vi "ConfigInstr.vi"(6 "InstrumentName":string, 7 "VisaRessIn":refnum<visa-resource-name>, 8 "error in (no error)":errorcluster caption="entrée d'erreur (pas d'erreur)", 9 "FirstClassInst":bool, 10 "Function":string, 11 "GenData In":refnum<class "AppliedMotionDrive.lvclass"> caption="DNL_LabVIEW Object in") -> (0 "error out":errorcluster caption="sortie d'erreur", 3 "GenData Out":refnum<class "AppliedMotionDrive.lvclass"> caption="DNL_LabVIEW Object out")   [LabVIEW 2019, in "AppliedMotionDrive.lvclass"]
uses:
  AppliedMotionDrive.lvclass
  C:/Programmes Labview/LabscanV1A/DevicesClass/BaseDevice/BaseDevice.lvclass
  AppliedMotionDrive_Func.ctl
  AppliedMotionDrive.lvclass/AppliedMotionDrive.ctl
  BaseDevice/BaseDevice.lvclass/BaseDevice.ctl
  BaseDevice/Accessor/SetShowInstrNm.vi
  BaseDevice/Accessor/SetInstrParam.vi
panel:
  in  "DefaultDev_Func":T1
  out "VisaRessOut":refnum<visa-resource-name>
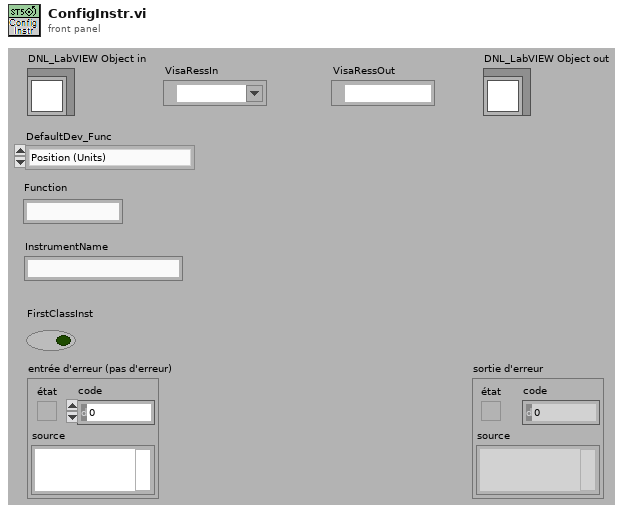
[diagram p1: front panel]
types:
  T1 = typedef "AppliedMotionDrive.lvclass/AppliedMotionDrive_Func.ctl" = enum16{"Position (Units)", "FilterWheel (Id)"}
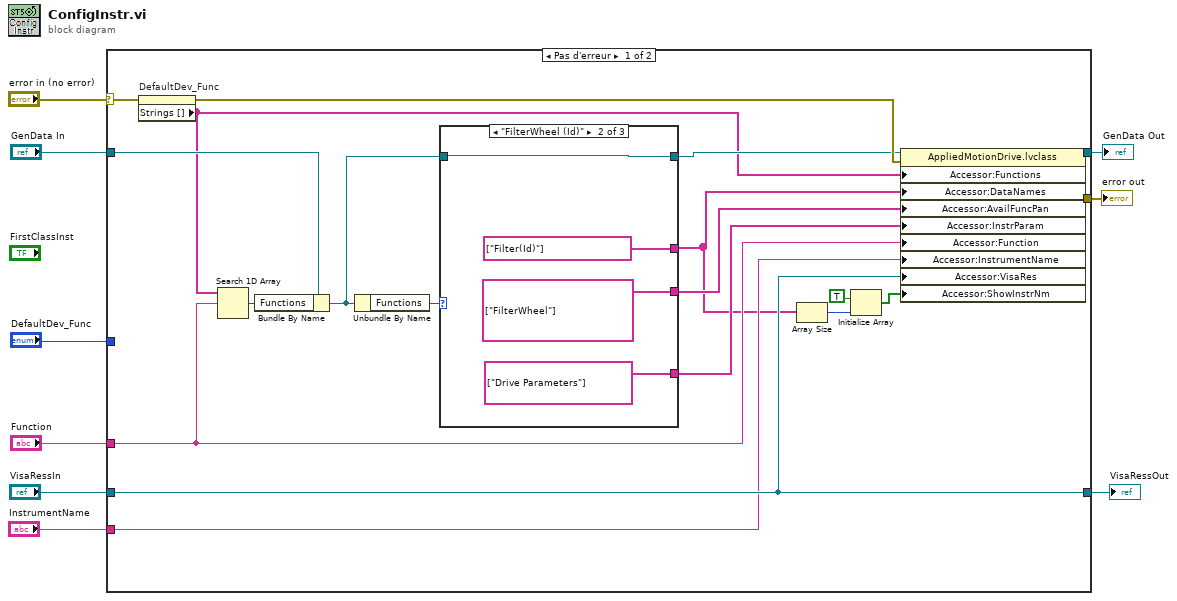
[diagram p0: block diagram]
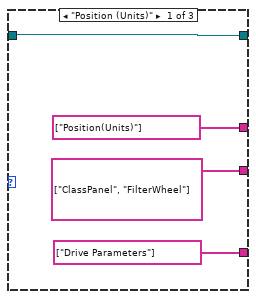
[diagram p2: hidden frame]
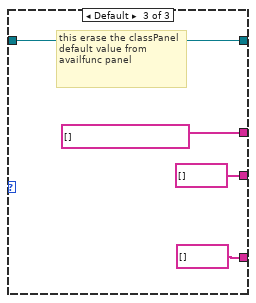
[diagram p3: hidden frame]
diagram:
  n1 = case shown="Pas d'erreur" "error in (no error)" {
    selector: "error in (no error)" -> [w24 w43]
    tunnel: [w28 w43] -> w8
    tunnel: "GenData In" -> [w19 w42]
    tunnel: [w27 w42] -> w6
    tunnel: "DefaultDev_Func" -> [_ _]
    tunnel: "Function" -> [w15 _]
    tunnel: "InstrumentName" -> [w17 _]
    tunnel: "VisaRessIn" -> [w20 w41]
    tunnel: [w20 w41] -> w1
    frame No Error {
      n2 = property on="DefaultDev_Func" class="Énum (strict)"(error in=w24) -> (error out=w23:errorcluster, "Strings []"=w16:string[])  [unwired: 1 in, 1 out]
      n3 = Search 1D Array(1D array=w16, element=w15) -> (index of element=w25:i32)  [unwired: 1 in]
      n4 = Bundle By Name(cluster=w19, "Functions"=w25) -> (w22:refnum<class "AppliedMotionDrive.lvclass">)
      n5 = Unbundle By Name(w22) -> ("Functions"=w26:T1)
      n6 = case shown="\"FilterWheel (Id)\"" w26 {
        tunnel: [string[] ["Position(Units)"] string[] ["Filter(Id)"] string[] []] -> w10
        tunnel: w22 -> [w32 w36 w39]
        tunnel: [w32 w36 w39] -> w21
        tunnel: [string[] ["ClassPanel", "FilterWheel"] string[] ["FilterWheel"] string[] []] -> w18
        tunnel: [string[] ["Drive Parameters"] ("InstrParam") string[] ["Drive Parameters"] ("InstrParam") string[] []] -> w14
        frame "Position (Units)" {
        }
        frame "FilterWheel (Id)" {
        }
        frame Default {
          # "this erase the classPanel default value from availfunc panel"
        }
      }
      n7 = Array Size(array=w10) -> (size(s)=w13:i32)
      n8 = Initialize Array(TRUE, w13) -> (w11:bool[])
      n9 = property class="AppliedMotionDrive.lvclass"(reference=w21, error in=w23, "Accessor:Functions"=w16, "Accessor:DataNames"=w10, "Accessor:AvailFuncPan"=w18, "Accessor:InstrParam"=w14, "Accessor:Function"=w15, "Accessor:InstrumentName"=w17, "Accessor:VisaRes"=w20, "Accessor:ShowInstrNm"=w11) -> (reference out=w27:refnum<class "AppliedMotionDrive.lvclass">, error out=w28:errorcluster)
    }
    frame Error {
    }
  }
  "error out" <- w8
  "GenData Out" <- w6
  "VisaRessOut" <- w1
